vi "New File (4-28-20220).vi"   [LabVIEW 2020]
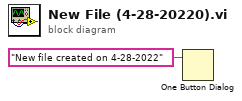
[diagram p0: block diagram]
diagram:
  n1 = One Button Dialog(message="New file created on 4-28-2022") -> ()  [unwired: 1 in, 1 out]
